vi "Parse Input Signals.vi"(8 "error in (no error)":errorcluster, 11 "Device Reference in":T3 format="%.0x") -> (0 "error out":errorcluster, 1 "Input Signals":refnum<k21>[](array[refnum]), 2 "Block Data Refs":T1[](array[typedef]) {"Data Reference" format="%.0x"}, 3 "Device Ref out":T3 format="%.0x", 5 "Output Values":dbl[](array[numeric]))   [LabVIEW 2009, in "NI-XNET Custom Device.lvlib"]
doc: "This VI is used to parse out all the NI-XNET input signals information from the system explorer tree. Here, we get a list of NI-XNET signals names that will be used to create an input session."
uses:
  NI-XNET Custom Device.lvlib
  <vilib>/NI VeriStand/Custom Device API/Custom Device Item Ref.ctl
  <vilib>/NI VeriStand/Custom Device API/Block Data Reference.ctl
  <vilib>/NI VeriStand/Custom Device API/Data Reference.ctl
  <vilib>/NI VeriStand/Custom Device API/Custom Device Channel Type.ctl
  <vilib>/NI VeriStand/Custom Device API/Data Access Type.ctl
  <vilib>/NI VeriStand/Custom Device API/Get Item Property (Variant).vi
  <vilib>/NI VeriStand/Custom Device API/Custom Device API.lvlib
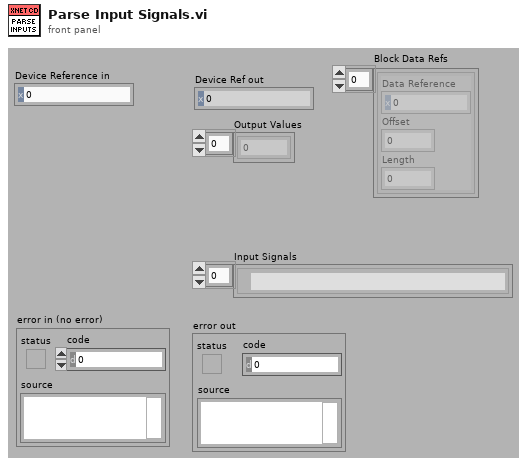
[diagram p1: front panel]
types:
  T1 = typedef "Custom Device API.lvlib/Block Data Reference.ctl" = cluster{"Data Reference":T2, "Offset":i32, "Length":i32}
  T2 = typedef "Custom Device API.lvlib/Data Reference.ctl" = i32
  T3 = typedef "Custom Device API.lvlib/Custom Device Item Ref.ctl" = u64
  T4 = typedef "Custom Device API.lvlib/Data Access Type.ctl" = enum16{"Read", "Write"}
  T5 = typedef "Custom Device API.lvlib/Custom Device Channel Type.ctl" = enum16{"Input", "Output"}
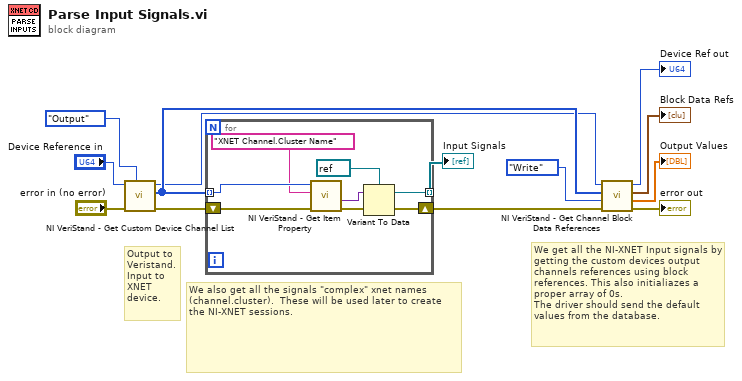
[diagram p0: block diagram]
diagram:
  # "We also get all the signals \"complex\" xnet names (channel.cluster).  These will be used later to create the NI-XNET sessions."
  # "We get all the NI-XNET Input signals by getting the custom devices output channels references using block references. This also initialiazes a proper array of 0s.\nThe driver should send the default values from the database."
  # "Output to Veristand.  Input to XNET device."
  n1 = call <vilib>:"NI VeriStand - Get Custom Device Channel List.vi"("Channel Type"=Custom_Device_Channel_Type."Output", "error in (no error)"="error in (no error)", "Device Ref in"="Device Reference in") -> ("error out"=w11:errorcluster, "Specified Channel Ref List"=w6:T3[], "Device Ref out"=w3:T3)  [unwired: 6 out]
  n2 = for {
    tunnel: w6 -> [w21] mode=indexing
    shift-right: [w19] -> w1
    shift-left: w11 -> [w14]
    tunnel: [w20] -> w12 mode=indexing
    n3 = call-poly <vilib>:"NI VeriStand - Get Item Property.vi"("error in (no error)"=w14, "Property Name"="XNET Channel.Cluster Name", "Item Ref in"=w21) -> ("error out"=w15:errorcluster, "Value"=w16:variant)  [unwired: 5 in, 2 out]
    n4 = Variant To Data(error in=w15, Variant=w16, type=refnum<k21> refnum ("XNET Signal")) -> (error out=w19:errorcluster, data=w20:refnum<k21>)
  }
  "Input Signals" <- w12
  n5 = call <vilib>:"NI VeriStand - Get Channel Block Data References.vi"("error in (no error)"=w1, "Access"=Data_Access_Type."Write", "Channel Refs"=w6, "Device Ref in"=w3) -> ("error out"=→"error out":errorcluster, "Values Array"=→"Output Values":dbl[], "Block Data Refs"=→"Block Data Refs":T1[], "Device Ref out"=→"Device Ref out":T3)  [unwired: 4 out]
